vi "Read Power Measurements.vi"(0 "VISA resource name":refnum<visa-resource-name>, 11 "error in (no error)":errorcluster) -> (2 "Actual Real Power (W)":dbl format="%.4g", 3 "Actual Apparent Power (VA)":dbl format="%.4g", 4 "VISA resource name out":refnum<visa-resource-name>, 6 "Actual Reactive Power (VAR)":dbl format="%.4g", 8 "Actual Power Factor":dbl format="%.4g", 10 "Actual Inrush Current (A)":dbl format="%.4g", 13 "Actual Negative Current Peak (Apk)":dbl format="%.4g", 14 "Actual Positive Current Peak (Apk)":dbl format="%.4g", 15 "error out":errorcluster)   [LabVIEW 2015, in "BK Precision 983X Series.lvlib"]
doc: "Measures the AC real, apparent, and reactive power, power factor, peak current, and inrush current of the output."
uses:
  <instrlib>/BK Precision 983X Series/BK Precision 983X Series.lvlib
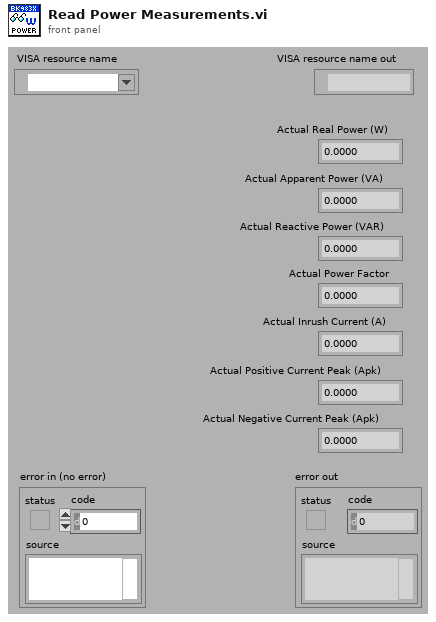
[diagram p1: front panel]
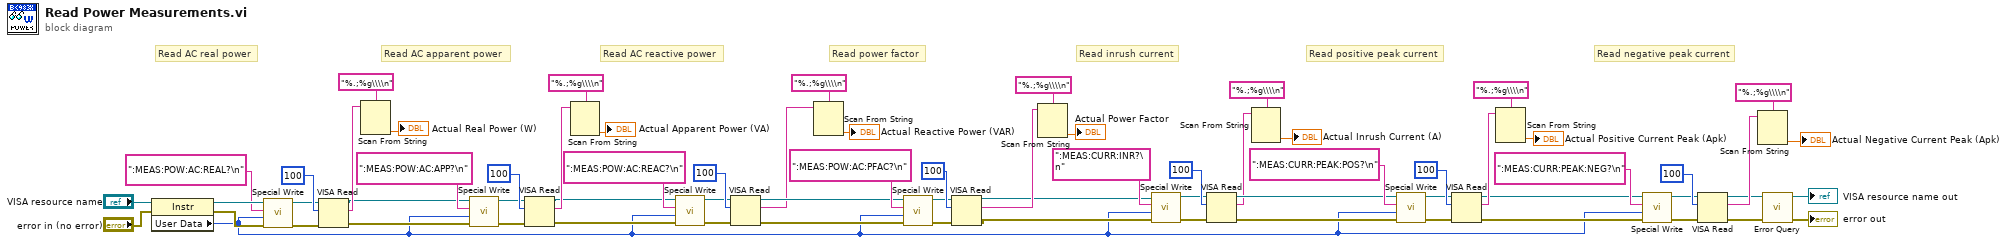
[diagram p0: block diagram]
diagram:
  # "Read negative peak current"
  # "Read positive peak current"
  # "Read inrush current"
  # "Read power factor"
  # "Read AC reactive power"
  # "Read AC apparent power"
  # "Read AC real power"
  n1 = property class="Instr"(reference="VISA resource name", error in="error in (no error)") -> (reference out=w59:refnum<visa-resource-name>, error out=w60:errorcluster, "User Data"=w5:u32)
  n2 = call <instrlib>:"Special Write.vi"("error in (no error)"=w60, "Delay (0 ms)"=w5, "Input String"=":MEAS:POW:AC:REAL?\n", "VISA resource name"=w59) -> ("error out"=w63:errorcluster, "VISA resource name out"=w64:refnum<visa-resource-name>)  [unwired: 6 in]
  n3 = VISA Read(VISA resource name=w64, byte count=u32 100, error in (no error)=w63) -> (VISA resource name out=w33:refnum<visa-resource-name>, read buffer=w67:string, error out=w32:errorcluster)  [unwired: 1 out]
  n4 = Scan From String(format string="%.;%g\\\\n", input string=w67) -> (output 1=→"Actual Real Power (W)":dbl)  [unwired: 3 in, 3 out]
  n5 = call <instrlib>:"Special Write.vi"("error in (no error)"=w32, "Delay (0 ms)"=w5, "Input String"=":MEAS:POW:AC:APP?\n", "VISA resource name"=w33) -> ("error out"=w55:errorcluster, "VISA resource name out"=w56:refnum<visa-resource-name>)  [unwired: 6 in]
  n6 = VISA Read(VISA resource name=w56, byte count=u32 100, error in (no error)=w55) -> (VISA resource name out=w29:refnum<visa-resource-name>, read buffer=w30:string, error out=w28:errorcluster)  [unwired: 1 out]
  n7 = Scan From String(format string="%.;%g\\\\n", input string=w30) -> (output 1=→"Actual Apparent Power (VA)":dbl)  [unwired: 3 in, 3 out]
  n8 = call <instrlib>:"Special Write.vi"("error in (no error)"=w28, "Delay (0 ms)"=w5, "Input String"=":MEAS:POW:AC:REAC?\n", "VISA resource name"=w29) -> ("error out"=w51:errorcluster, "VISA resource name out"=w52:refnum<visa-resource-name>)  [unwired: 6 in]
  n9 = VISA Read(VISA resource name=w52, byte count=u32 100, error in (no error)=w51) -> (VISA resource name out=w27:refnum<visa-resource-name>, read buffer=w24:string, error out=w26:errorcluster)  [unwired: 1 out]
  n10 = Scan From String(format string="%.;%g\\\\n", input string=w24) -> (output 1=→"Actual Reactive Power (VAR)":dbl)  [unwired: 3 in, 3 out]
  n11 = call <instrlib>:"Special Write.vi"("error in (no error)"=w26, "Delay (0 ms)"=w5, "Input String"=":MEAS:POW:AC:PFAC?\n", "VISA resource name"=w27) -> ("error out"=w47:errorcluster, "VISA resource name out"=w48:refnum<visa-resource-name>)  [unwired: 6 in]
  n12 = VISA Read(VISA resource name=w48, byte count=u32 100, error in (no error)=w47) -> (VISA resource name out=w20:refnum<visa-resource-name>, read buffer=w23:string, error out=w21:errorcluster)  [unwired: 1 out]
  n13 = Scan From String(format string="%.;%g\\\\n", input string=w23) -> (output 1=→"Actual Power Factor":dbl)  [unwired: 3 in, 3 out]
  n14 = call <instrlib>:"Special Write.vi"("error in (no error)"=w21, "Delay (0 ms)"=w5, "Input String"=":MEAS:CURR:INR?\n", "VISA resource name"=w20) -> ("error out"=w43:errorcluster, "VISA resource name out"=w44:refnum<visa-resource-name>)  [unwired: 6 in]
  n15 = VISA Read(VISA resource name=w44, byte count=u32 100, error in (no error)=w43) -> (VISA resource name out=w19:refnum<visa-resource-name>, read buffer=w17:string, error out=w18:errorcluster)  [unwired: 1 out]
  n16 = Scan From String(format string="%.;%g\\\\n", input string=w17) -> (output 1=→"Actual Inrush Current (A)":dbl)  [unwired: 3 in, 3 out]
  n17 = call <instrlib>:"Special Write.vi"("error in (no error)"=w18, "Delay (0 ms)"=w5, "Input String"=":MEAS:CURR:PEAK:POS?\n", "VISA resource name"=w19) -> ("error out"=w39:errorcluster, "VISA resource name out"=w40:refnum<visa-resource-name>)  [unwired: 6 in]
  n18 = VISA Read(VISA resource name=w40, byte count=u32 100, error in (no error)=w39) -> (VISA resource name out=w7:refnum<visa-resource-name>, read buffer=w9:string, error out=w6:errorcluster)  [unwired: 1 out]
  n19 = Scan From String(format string="%.;%g\\\\n", input string=w9) -> (output 1=→"Actual Positive Current Peak (Apk)":dbl)  [unwired: 3 in, 3 out]
  n20 = call <instrlib>:"Special Write.vi"("error in (no error)"=w6, "Delay (0 ms)"=w5, "Input String"=":MEAS:CURR:PEAK:NEG?\n", "VISA resource name"=w7) -> ("error out"=w11:errorcluster, "VISA resource name out"=w12:refnum<visa-resource-name>)  [unwired: 6 in]
  n21 = VISA Read(VISA resource name=w12, byte count=u32 100, error in (no error)=w11) -> (VISA resource name out=w2:refnum<visa-resource-name>, read buffer=w4:string, error out=w1:errorcluster)  [unwired: 1 out]
  n22 = Scan From String(format string="%.;%g\\\\n", input string=w4) -> (output 1=→"Actual Negative Current Peak (Apk)":dbl)  [unwired: 3 in, 3 out]
  n23 = call <instrlib>:"Error Query.vi"("error in (no error)"=w1, "VISA resource name"=w2) -> ("error out"=→"error out":errorcluster, "VISA resource name out"=→"VISA resource name out":refnum<visa-resource-name>)  [unwired: 6 in, 2 out]
